vi "Drive Teleop.vi"(6 "Quick Turn":bool, 7 "Auto Align":bool, 10 "Wheel":dbl, 11 "Throttle":dbl) -> ()   [LabVIEW 2019]
uses:
  <vilib>/Rock Robotics/Network Tables/NT Write Number.vi
  <vilib>/Rock Robotics/Network Tables/NT Read Number.vi
  Framework/Robot Global Data.vi
panel:
  in  "Deadband Value":dbl=0.01
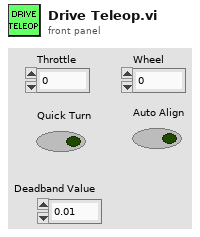
[diagram p1: front panel]
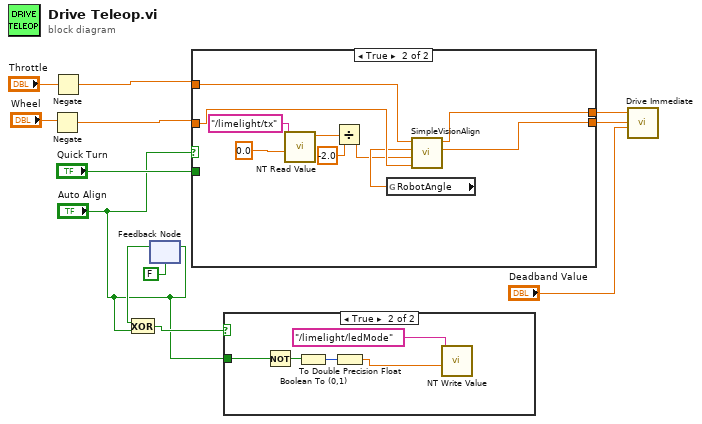
[diagram p0: block diagram]
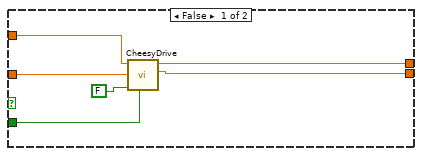
[diagram p3: hidden frame]
diagram:
  n1 = Negate(x="Wheel") -> (-x=w2:dbl)
  n2 = Negate(x="Throttle") -> (-x=w1:dbl)
  n3 = feedback-in #1("Auto Align") -> ()
  n4 = feedback #1(FALSE) -> (w5:bool)
  n5 = Exclusive Or(1:"Auto Align", 2:w5) -> (0:w4:bool)
  n6 = case shown="True" "Auto Align" {
    tunnel: w1 -> [w18 w25]
    tunnel: w2 -> [w17 w26]
    tunnel: "Quick Turn" -> [w16 _]
    tunnel: [w14 w24] -> w11
    tunnel: [w13 w23] -> w10
    frame False {
      n7 = call "CheesyDrive.vi"("Quickturn"=w16, "Fast Mode"=FALSE, "Wheel"=w17, "Throttle"=w18) -> ("Right PWM"=w13:dbl, "Left PWM"=w14:dbl)  [unwired: 6 in]
    }
    frame True {
      n8 = call-poly <vilib>:"NT Read Value.vi"("Default Value"=0.0, "Name"="/limelight/tx") -> ("Numeric"=w21:dbl)  [unwired: 8 in, 1 out]
      n9 = Divide(x=w21, y=-2.0) -> (x/y=w19:dbl)
      n10 = global read "Robot Global Data.vi" "RobotAngle"() -> (w22:dbl)
      n11 = call "SimpleVisionAlign.vi"("Manual Turn"=w26, "Target Offset"=w19, "Gyro Angle"=w22, "Throttle"=w25) -> ("Right Power"=w23:dbl, "Left Power"=w24:dbl)  [unwired: 6 in]
    }
  }
  n12 = case shown="True" w4 {
    tunnel: "Auto Align" -> [_ w33]
    frame False {
    }
    frame True {
      n13 = Not(x=w33) -> (.not. x?=w32:bool)
      n14 = Boolean To (0,1)(Boolean=w32) -> (0, 1=w30:i16)
      n15 = To Double Precision Float(number=w30) -> (double precision float=w29:dbl)
      n16 = call-poly <vilib>:"NT Write Value.vi"("Numeric"=w29, "Name"="/limelight/ledMode") -> ()  [unwired: 9 in, 1 out]
    }
  }
  n17 = call "Drive Immediate.vi"("Deadband Value"="Deadband Value", "Right Setpoint"=w10, "Left Setpoint"=w11) -> ()  [unwired: 8 in, 1 out]
